vi "Clear TCP AI.vi"(8 "error in (no error)":errorcluster, 11 "Connection ID in":refnum<k5>) -> (0 "error out":errorcluster, 3 "Connection ID out":refnum<k5>)   [LabVIEW 2019]
doc: "This VI sends the idle command to the data server and attempts to clear any data in the TCP buffers with a long read.\n\nInputs\n\nConnection ID in - TCP connection\n\nerror in - \n\nOutputs\n\nConnection ID out - TCP connection\n\nerror out - \n\nCreated by Monroe Weber-Shirk\nCornell University\nmw24@cornell.edu\nJanuary 2000"
uses:
  DataServer/command.ctl
  DataServer/command cluster.ctl
panel:
  in  "command interface":T1={"command"=enum."Idle", "start time (ms)"=0, "Channel Indices"=[], "Scans per Sample"=1} {"Scans per Sample" min=1}
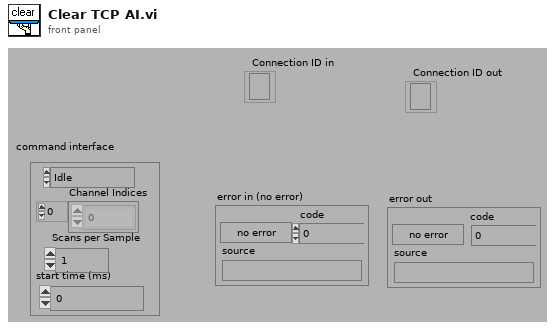
[diagram p1: front panel]
types:
  T1 = typedef "command cluster.ctl" = cluster{"command":T2, "start time (ms)":u32, "Channel Indices":i32[], "Scans per Sample":i32}
  T2 = typedef "command.ctl" = enum16{"Idle", "Send Data", "Send 1 Scan", "Logoff"}
  T3 = enum16{"Standard", "Buffered", "CRLF", "Immediate"}
  T4 = enum16{"Idle", "Send Data", "Send 1 Scan", "Logoff"}
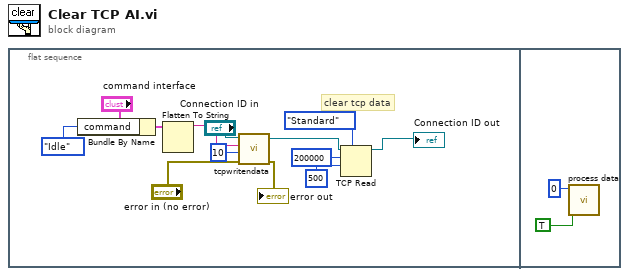
[diagram p0: block diagram]
diagram:
  n1 = flat-sequence {
    frame #0 {
      # "clear tcp data"
      n2 = Bundle By Name(cluster="command interface", "command"=T4."Idle") -> (w9:T1)
      n3 = Flatten To String(anything=w9) -> (data string=w11:string)  [unwired: 3 in, 2 out]
      n4 = call "tcpwritendata.vi"("error in (no error)"="error in (no error)", "timeout ms (25000)"=10, "data in"=w11, "refnum in"="Connection ID in") -> ("error out"=→"error out":errorcluster, "refnum out"=w7:refnum<k5>)  [unwired: 5 in, 1 out]
      n5 = TCP Read(connection ID=w7, bytes to read=200000, 7:T3."Standard" ("mode (standard)"), 9:500 ("timeout ms (25000)")) -> (connection ID out=→"Connection ID out":refnum<k5>)  [unwired: 1 in, 2 out]
    }
    frame #1 {
      n6 = call "process data.vi"("Reset"=TRUE, "successes"=u32 0) -> ()  [unwired: 6 in, 4 out]
    }
  }
